vi "lab1.vi"() -> ()   [LabVIEW 2014]
panel:
  out "Array":i32[][](array[numeric])
  in  "n-step":i32
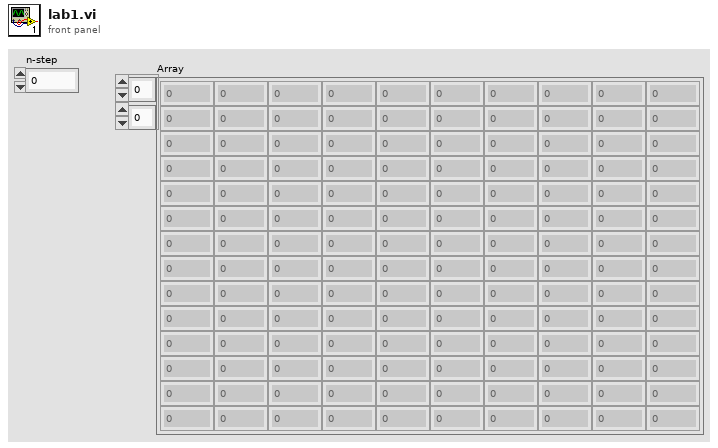
[diagram p1: front panel]
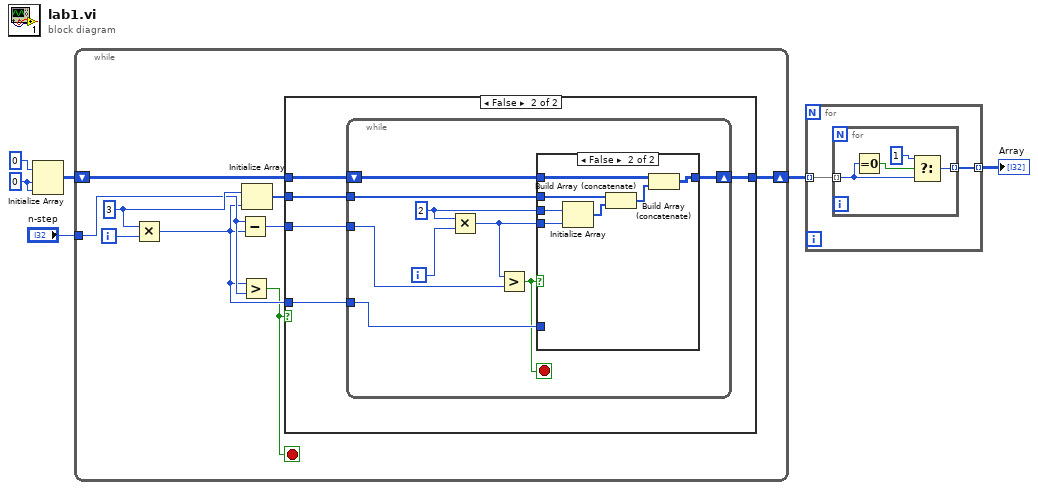
[diagram p0: block diagram]
diagram:
  w3 = 0 ("dimension size")
  n1 = Initialize Array(0 ("element"), w3, w3) -> (w6:i32[][])
  n2 = while {
    tunnel: "n-step" -> [w12]
    shift-right: [w9] -> w2
    shift-left: w6 -> [w10]
    i -> [w15]
    stop <- w7 stop-if-true
    w14 = 3 ("y")
    n3 = Multiply(x=w14, y=w15) -> (x*y=w11:i32)
    n4 = Subtract(x=w12, y=w11) -> (x-y=w8:i32)
    n5 = Greater?(x=w11, y=w12) -> (0:w7:bool)
    n6 = Initialize Array(w14, w11) -> (w13:i32[])
    n7 = case shown="False" w7 {
      tunnel: w13 -> [_ w21]
      tunnel: w8 -> [_ w20]
      tunnel: w11 -> [_ w19]
      tunnel: w10 -> [w16 w18]
      tunnel: [w16 w17] -> w9
      frame True {
      }
      frame False {
        n8 = while {
          tunnel: w21 -> [w27]
          tunnel: w20 -> [w23]
          tunnel: w19 -> [w26]
          shift-right: [w24] -> w17
          shift-left: w18 -> [w25]
          i -> [w30]
          stop <- w22 stop-if-true
          w29 = 2 ("y")
          n9 = Multiply(x=w29, y=w30) -> (x*y=w28:i32)
          n10 = Greater?(x=w28, y=w23) -> (0:w22:bool)
          n11 = case shown="False" w22 {
            tunnel: w29 -> [_ w38]
            tunnel: w28 -> [_ w37]
            tunnel: w27 -> [_ w36]
            tunnel: w26 -> [_ _]
            tunnel: w25 -> [w31 w33]
            tunnel: [w31 w32] -> w24
            frame True {
            }
            frame False {
              n12 = Initialize Array(w38, w37) -> (w35:i32[])
              n13 = Build Array (concatenate)(w36, w35) -> (w34:i32[])
              n14 = Build Array (concatenate)(w33, w34) -> (w32:i32[][])
            }
          }
        }
      }
    }
  }
  n15 = for {
    tunnel: w2 -> [w40] mode=indexing
    tunnel: [w39] -> w1 mode=indexing
    n16 = for {
      tunnel: w40 -> [w42] mode=indexing
      tunnel: [w41] -> w39 mode=indexing
      n17 = Equal To 0?(x=w42) -> (x = 0?=w44:bool)
      n18 = Select(t=1 ("y"), s=w44, f=w42) -> (s? t:f=w41:i32)
    }
  }
  "Array" <- w1
